vi "CheckData.vi"(5 "Queue Cluster":T1, 7 "DATA":i16[](array[numeric]), 8 "error in (no error)":errorcluster, 11 "Process in":refnum<class "Process.lvclass">) -> (0 "error out":errorcluster, 3 "Process out":refnum<class "Process.lvclass">)   [LabVIEW 2017, in "Process.lvclass"]
uses:
  Process.lvclass
  Ctl/MEMS.ctl
  ModbusRTUCmd.ctl
  Process.ctl
  Caculator/Caculator.ctl
  Process.lvclass/Process.ctl
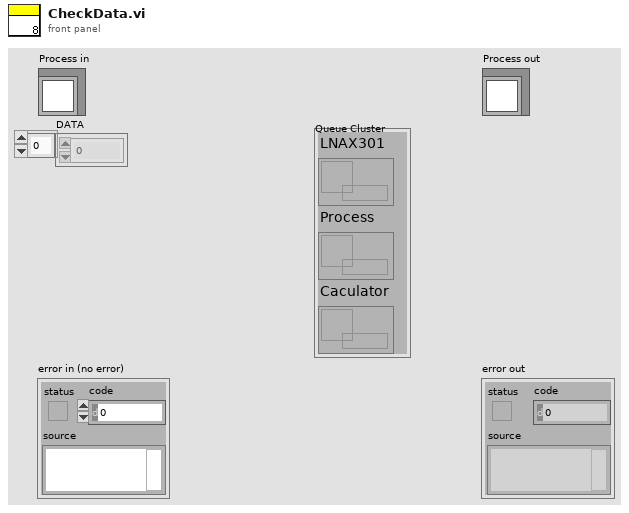
[diagram p1: front panel]
types:
  T1 = typedef "MEMS.ctl" = cluster{"LNAX301":refnum<queue>, "Process":refnum<queue>, "Caculator":refnum<queue>}
  T2 = typedef "Caculator.ctl" = cluster{"cmd":enum16{"Idle", "ini", "Disconnect", "UpdateSetup", "ChangeView", "Caculator", "Exit"}, "Var":variant}
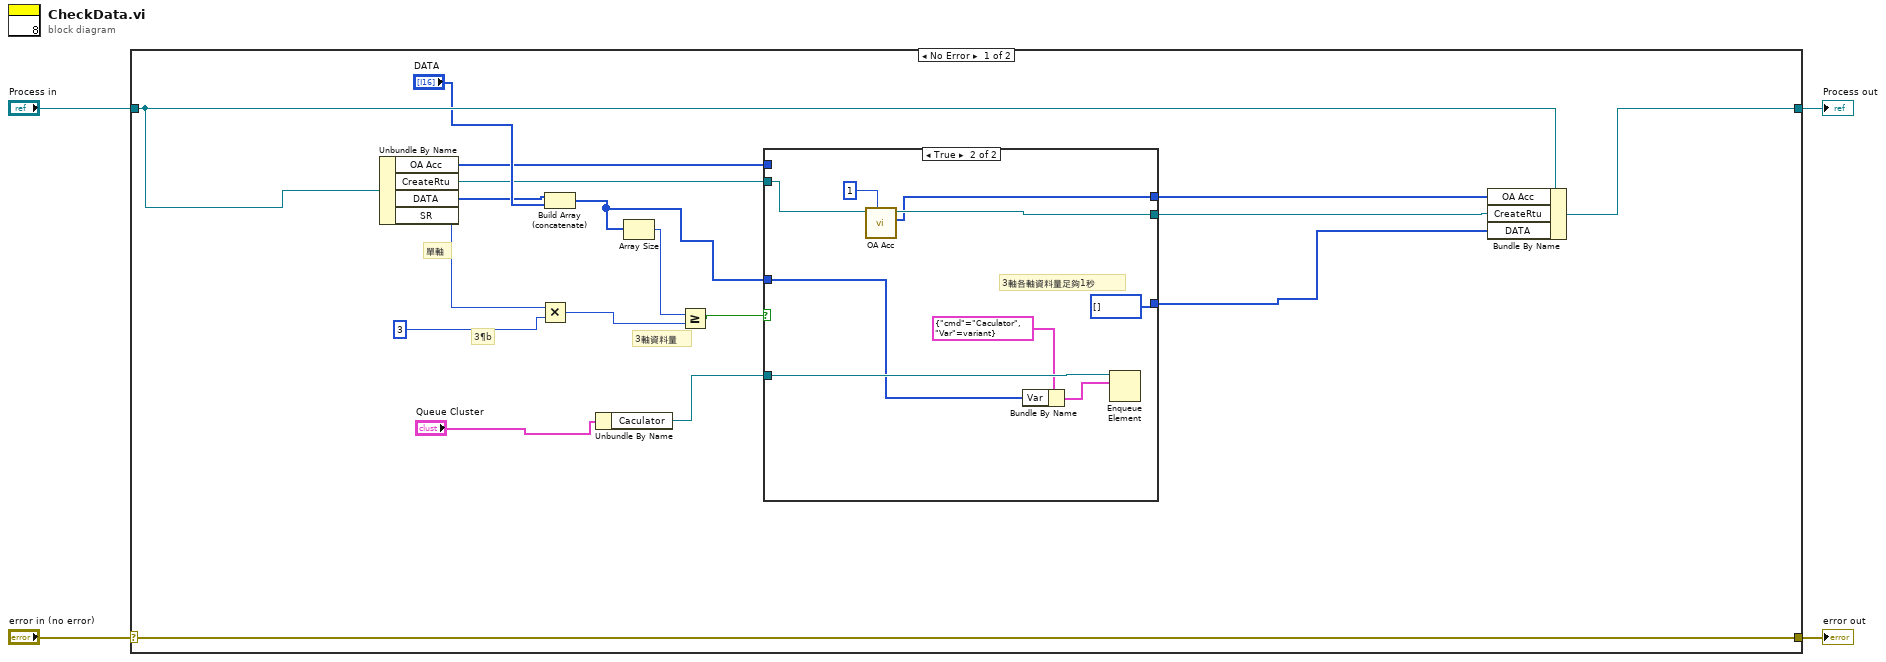
[diagram p0: block diagram]
diagram:
  n1 = case shown="No Error" "error in (no error)" {
    selector: "error in (no error)" -> [w22 w36]
    tunnel: [w22 w36] -> w3
    tunnel: [w15 w35] -> w1
    tunnel: "Process in" -> [w21 w35]
    frame No Error {
      # "3軸資料量"
      # "3¶b"
      # "單軸"
      n2 = Unbundle By Name(w21) -> ("OA Acc"=w5:u16[], "CreateRtu"=w6:refnum<k24>, "DATA"=w9:i16[], "SR"=w13:u16)
      n3 = Multiply(x=w13, y=u16 3) -> (x*y=w10:u16)
      n4 = Build Array (concatenate)(w9, "DATA") -> (w8:i16[])
      n5 = Unbundle By Name("Queue Cluster") -> ("Caculator"=w18:refnum<queue>)
      n6 = Array Size(array=w8) -> (size(s)=w11:i32)
      n7 = Greater Or Equal?(x=w11, y=w10) -> (x >= y?=w7:bool)
      n8 = case shown="True" w7 {
        tunnel: w8 -> [w25 w30]
        tunnel: w18 -> [_ w34]
        tunnel: [w25 i16[] []] -> w17
        tunnel: w6 -> [w24 w29]
        tunnel: [w24 w27] -> w16
        tunnel: [w23 w26] -> w14
        tunnel: w5 -> [w23 _]
        frame False {
        }
        frame True {
          # "3軸各軸資料量足夠1秒"
          n9 = call "OA Acc.vi"("SlaveID"=u8 1, ".NET Refnum in"=w29) -> ("OA Acc"=w26:u16[], "reference out"=w27:refnum<k24>)  [unwired: 7 in, 1 out]
          n10 = Bundle By Name(cluster=T2 {"cmd"=enum."Caculator", "Var"=variant} ("element"), "Var"=w30) -> (w32:T2)
          n11 = Enqueue Element(queue=w34, element=w32) -> ()  [unwired: 2 in, 3 out]
        }
      }
      n12 = Bundle By Name(cluster=w21, "OA Acc"=w14, "CreateRtu"=w16, "DATA"=w17) -> (w15:refnum<class "Process.lvclass">)
    }
    frame Error {
    }
  }
  "error out" <- w3
  "Process out" <- w1
